vi "Bairstow_Calculate B_C.vi"(9 "r":dbl, 10 "s":dbl, 11 "P(x)":dbl[](array[numeric])) -> (2 "C":dbl[](array[numeric]), 3 "B":dbl[](array[numeric]))   [LabVIEW 2017, in "NI_AALPro.lvlib"]
uses:
  NI_AALPro.lvlib
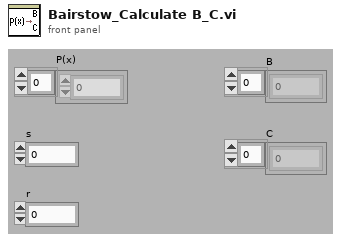
[diagram p1: front panel]
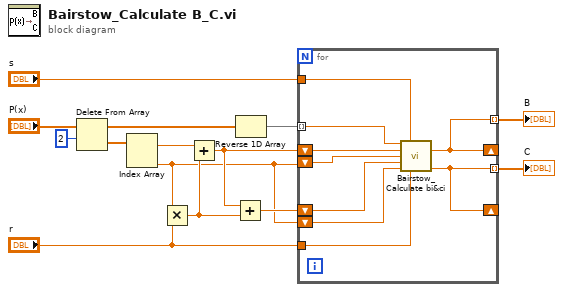
[diagram p0: block diagram]
diagram:
  n1 = Delete From Array(array="P(x)", length=2) -> (deleted portion=w2:dbl[], array with subset deleted=w4:dbl[])  [unwired: 1 in]
  n2 = Index Array(array=w2) -> (element #1=w10:dbl, element #2=w6:dbl)  [unwired: 2 in]
  n3 = Multiply(x=w6, y="r") -> (x*y=w11:dbl)
  n4 = Add(x=w10, y=w11) -> (x+y=w8:dbl)
  n5 = Add(x=w8, y=w11) -> (x+y=w7:dbl)
  n6 = Reverse 1D Array(array=w4) -> (reversed array=w1:dbl[])
  n7 = for {
    shift-right: [w20] -> _
    shift-left: w8 -> [w16]
    shift-left: w6 -> [w17]
    tunnel: w1 -> [w21] mode=indexing
    shift-right: [w15] -> _
    shift-left: w7 -> [w18]
    shift-left: w6 -> [w19]
    tunnel: "s" -> [w23]
    tunnel: "r" -> [w22]
    tunnel: [w20] -> w13 mode=indexing
    tunnel: [w15] -> w12 mode=indexing
    n8 = call "Bairstow_Calculate bi&ci.vi"("a(i)"=w21, "s"=w23, "b(i+1)"=w16, "b(i+2)"=w17, "c(i+1)"=w18, "c(i+2)"=w19, "r"=w22) -> ("b(i)"=w20:dbl, "c(i)"=w15:dbl)  [unwired: 7 in]
  }
  "B" <- w13
  "C" <- w12
